vi "resetOutput.vi"(8 "error in (no error)":errorcluster, 11 "CQT_DDS in":refnum<class "CQT_DDS.lvclass">) -> (0 "error out":errorcluster, 3 "CQT_DDS out":refnum<class "CQT_DDS.lvclass">)   [LabVIEW 2009, in "Hardware.lvlib" / "Channels.lvlib" / "CQT_DDS.lvclass"]
uses:
  CQT_DDS.lvclass
  Generic/DDSOutput.lvclass
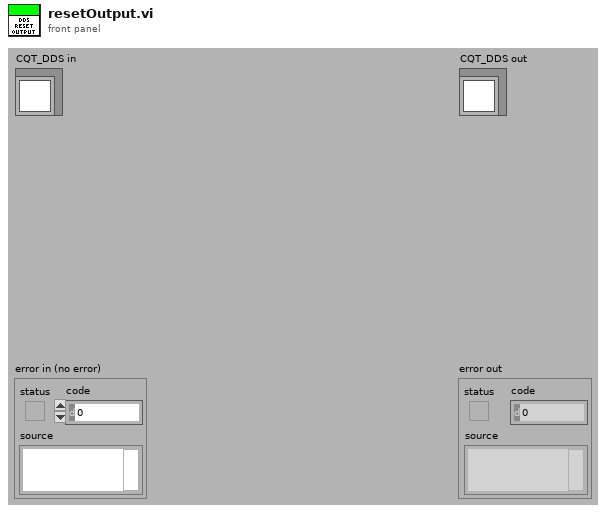
[diagram p1: front panel]
types:
  T1 = cluster{"Frequency(MHz)":dbl, "Amplitude":dbl, "Phase":dbl, "OutputForm":enum16{"Sine", "Square", "Triangle", "Arbitrary"}}[]
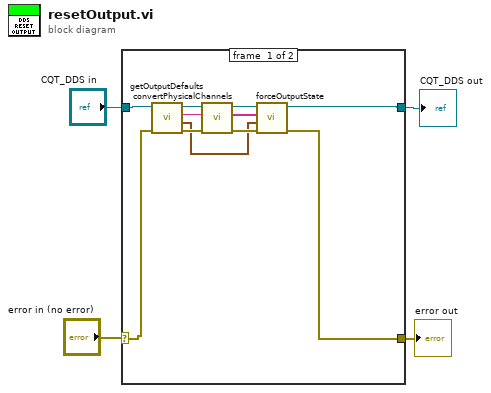
[diagram p0: block diagram]
diagram:
  n1 = case shown="No Error" "error in (no error)" {
    selector: "error in (no error)" -> [w14 w16]
    tunnel: [w5 w16] -> w3
    tunnel: [w6 w17] -> w2
    tunnel: "CQT_DDS in" -> [w15 w17]
    frame #0 {
      n2 = call "getOutputDefaults.vi"("error in (no error)"=w14, "DDSOutput in"=w15) -> ("error out"=w11:errorcluster, "Defaults"=w7:T1, "physical Channels"=w12:string, "DDSOutput out"=w13:refnum<class "CQT_DDS.lvclass">)  [unwired: 6 in]
      n3 = call "convertPhysicalChannels.vi"("error in (no error)"=w11, "physicalChannels"=w12, "DDSOutput in"=w13) -> ("error out"=w8:errorcluster, "physicalChannels"=w9:string[], "DDSOutput out"=w10:refnum<class "CQT_DDS.lvclass">)  [unwired: 6 in]
      n4 = call-dynamic "forceOutputState.vi"("error in (no error)"=w8, "data"=w7, "physicalChannels"=w9, "CQT_DDS in"=w10) -> ("error out"=w5:errorcluster, "CQT_DDS out"=w6:refnum<class "CQT_DDS.lvclass">)  [unwired: 6 in]
    }
    frame #1 {
    }
  }
  "error out" <- w3
  "CQT_DDS out" <- w2
